vi "Update Temperature.vi"(8 "error in (no error)":errorcluster, 10 "Temperature":dbl, 11 "Cooler UI with Events in":refnum<class "Cooler UI with Events.lvclass">) -> (0 "error out":errorcluster, 3 "Cooler UI with Events out":refnum<class "Cooler UI with Events.lvclass">)   [LabVIEW 2012, in "Cooler UI.lvlib" / "Cooler UI with Events.lvclass"]
uses:
  Cooler UI with Events.lvclass
  Cooler UI with Events.lvclass/Cooler UI with Events.ctl
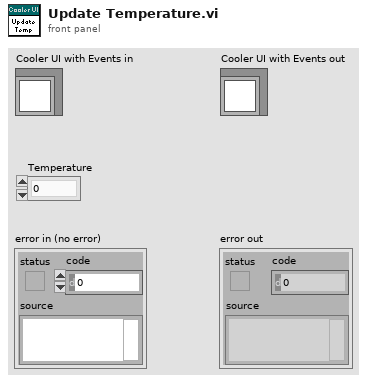
[diagram p1: front panel]
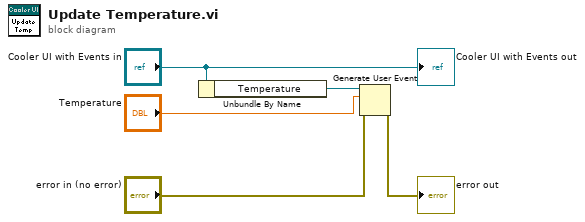
[diagram p0: block diagram]
diagram:
  n1 = Unbundle By Name("Cooler UI with Events in") -> ("Temperature"=w5:refnum<user-event>)
  n2 = Generate User Event(user event=w5, event data cluster="Temperature", error in="error in (no error)") -> (error out=→"error out":errorcluster)  [unwired: 1 out]
  "Cooler UI with Events out" <- "Cooler UI with Events in"
